vi "CRYUser Equation Parametes Table.vi"() -> ()   [LabVIEW 2013]
uses:
  Typedef Control/CRYUser Equation Cluster.ctl
  Typedef Control/CRYData Cluster Array.ctl
  Typedef Control/CRYData Cluster.ctl
  <vilib>/Utility/miscctls.llb/LVRowAndColumnTypeDef.ctl
  CRYPost Processing Global.vi
  CRYWindow/SubVI/CRYMain Sub Window Global.vi
panel:
  in  "DataNames":string[](array[string])
  in  "Curves&Values":T1 {"Z data" items=["dB", "Lin"]; "X data" items=["dB", "Lin"]; "Y data" items=["dB", "Lin"]; "Z dB ref" format="%.1f"; "Z axis" items=["Log", "Lin"]; "X dB ref" format="%.1f"; "X axis" items=["Log", "Lin"]; "Y axis" items=["Log", "Lin"]; "Y dB ref" format="%.1f"; "Curve"."z" format="%.2f"; "Curve"."y" format="%.2f"; "Curve"."x" format="%.2f"}
  in  "CurLibChange":bool caption="Add Lib"
  in  "On/Off Line":bool
  out "Clear All":bool
  out "In_Table Change":i32
  out "Res_Table Change":bool
  out "Row_unit res":i32
  out "User Equation Cluster":T3 {"Results axis" items=["x", "y", "z"]; "Input axis" items=["x", "y", "z"]; "Custom unit results array"."dB ref" format="%.2f"; "Custom unit input array"."dB ref" format="%.2f"}
  out "Load":bool
  out "String Ref Out":refnum<vi>
  out "Row_unit":i32
  in  "Unit_in":bool
  out "Row_axis":i32
  in  "Axis_Rnig":u16(ring) items=["x", "y", "z"]
  out "Row":i32
  in  "Ope_Ring":u16(ring) caption="Type" items=["<Select Operand>", "unity cal-in corr-in", "CRY33x Mic 1 corr-in", "CRY33x Mic 2 corr-in", "CRY33x Mic 3 corr-in", "CRY33x Mic 4 corr-in", "USB In L corr-in", "USB In R corr-in", "unity cal-out corr-out", "unity cal-out eq-out", "CRY602 Mouth 1 corr-out", "CRY602 Mouth 1 eq-out", "CRY602 Mouth 2 corr-out", "CRY602 Mouth 2 eq-out", "USB Out R corr-out", "USB Out R eq-out", "unity cal-in sens-in", "CRY33x Mic 1 sens-in", "CRY33x Mic 2 sens-in", "CRY33x Mic 3 sens-in", "CRY33x Mic 4 sens-in", "USB In L sens-in", "USB In R sens-in", "unity cal-out sens-out", "CRY602 Mouth 1 sens-out", "CRY602 Mouth 2 sens-out", "USB Out R sens-out", "User Defined Constant", "Remove this Item"]
  in  "stop":bool
  in  "Input_Table":string[][](table)
  in  "Unit_res":bool
  in  "Result_Table":string[][](table)
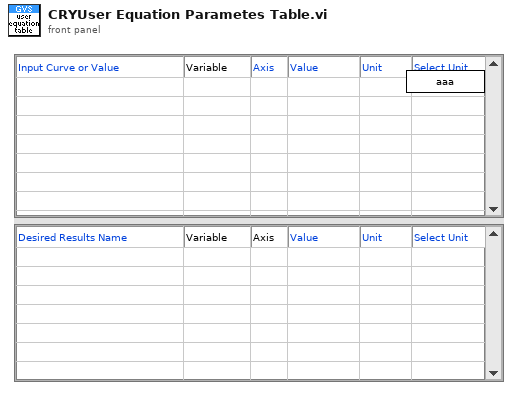
[diagram p1: front panel]
types:
  T1 = typedef "CRYData Cluster Array.ctl" = T2[]
  T2 = typedef "CRYData Cluster.ctl" = cluster{"Name":string, "Curve":cluster{"x":dbl, "y":dbl, "z":dbl}[], "X data":u16, "Y data":u16, "Z data":u16, "X axis":u16, "Y axis":u16, "Z axis":u16, "X unit":string, "Y unit":string, "Z unit":string, "X dB ref":dbl, "Y dB ref":dbl, "Z dB ref":dbl, "single val":bool, "protected":bool, "display X":bool, "display Y":bool, "display Z":bool, "Test Info":string, "Step No.":i32, "Plot Settings":cluster{"Color":u32, "Interpolation":u8, "Point Style":u8, "Line Style":u8, "Point Color":u32, "Line Width":u8, "Bar Plot Style":u8, "Fill To":i16}, "AutoProtect":bool}
  T3 = typedef "CRYUser Equation Cluster.ctl" = cluster{"Custom unit input array":cluster{"use custom":bool, "lin/log":u16, "unit":string, "dB ref":dbl, "common dB":u16}[], "Custom unit results array ":cluster{"use custom":bool, "lin/log":u16, "unit":string, "dB ref":dbl, "common dB":u16}[], "Desired Result Variables":string[], "Desired Result Names":string[], "Input Curve Names":string[], "Input Curve Variables":string[], "equation":string, "Input axis":u16[], "Results axis":u16[], "# input curves":i32, "# Desired result curves ":i32, "Input Values":string[], "Result Values":string[]}
  T4 = typedef "LVRowAndColumnTypeDef.ctl" = cluster{"Row":i32, "Column":i32}
  T5 = typedef "LVRectTypeDef.ctl" = cluster{"Left":i16, "Top":i16, "Right":i16, "Bottom":i16}
  T6 = typedef "CRYStep.ctl" = cluster{"No.VI":i32, "Category":string, "StepName":string, "Seq setup flattened":string, "Comment":string, "Steps config.":bool[], "Jump config":i32[], "Start":dbl, "Increment":dbl, "Name":string, "Unit":string, "Y data":u16, "Y prefix":string, "Y dB ref":dbl, "Y unit":string, "Repeat State Array":cluster{"Start":dbl, "Increment":dbl, "Count":i32, "Num":i32}[]}
  T7 = cluster{"use custom":bool, "lin/log":u16, "unit":string, "dB ref":dbl, "common dB":u16}
  T8 = enum16{"OK", "Yes", "YesNo", "YesNoCancel", "ReplaceAppend"}
  T9 = cluster{"use custom":bool, "lin/log":u16, "unit":string, "dB ref":dbl, "common dB":u16}[]
  T10 = typedef "LVPoint32TypeDef.ctl" = cluster{"Horizontal":i32, "Vertical":i32}
  T11 = typedef "LVBoundsTypeDef.ctl" = cluster{"Width":u32, "Height":u32}
  T12 = typedef "LVPositionTypeDef.ctl" = cluster{"Left":i32, "Top":i32}
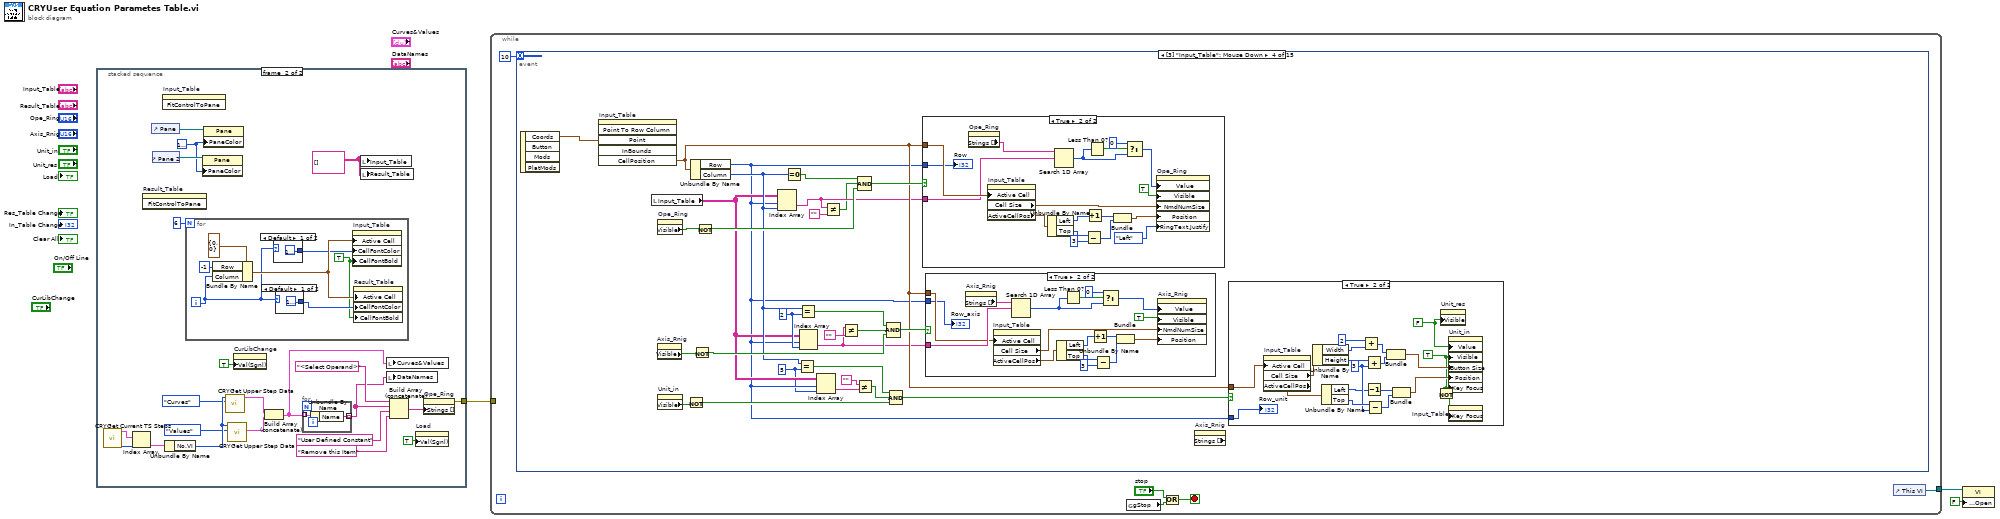
[diagram p0: block diagram]
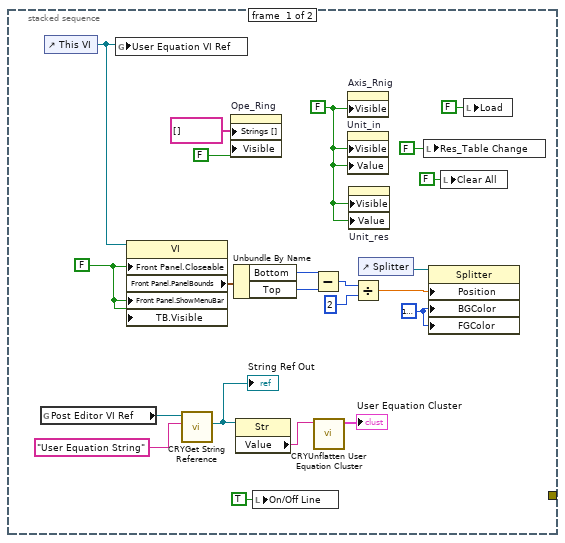
[diagram p2: hidden frame]
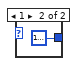
[diagram p3: hidden frame]
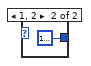
[diagram p4: hidden frame]
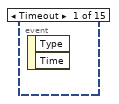
[diagram p5: hidden frame]
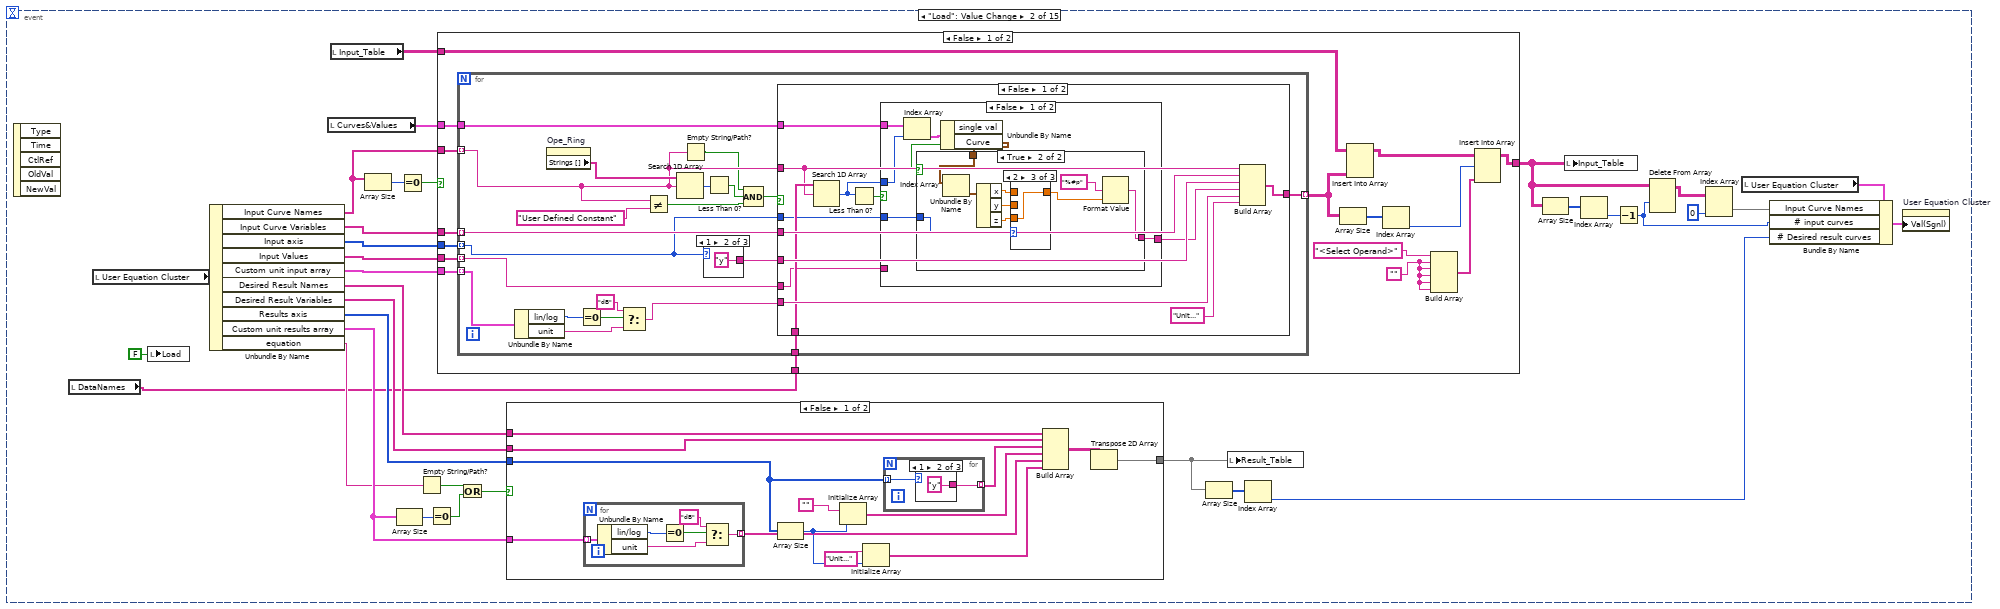
[diagram p6: hidden frame]
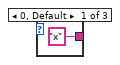
[diagram p7: hidden frame]
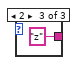
[diagram p8: hidden frame]
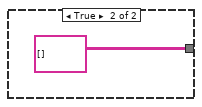
[diagram p9: hidden frame]
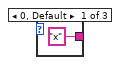
[diagram p10: hidden frame]
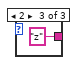
[diagram p11: hidden frame]
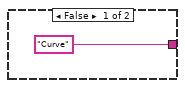
[diagram p12: hidden frame]
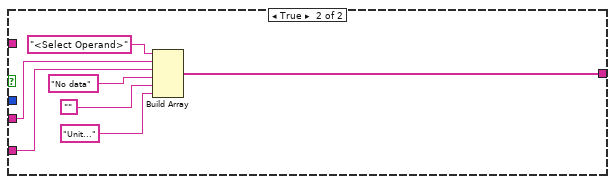
[diagram p16: hidden frame]
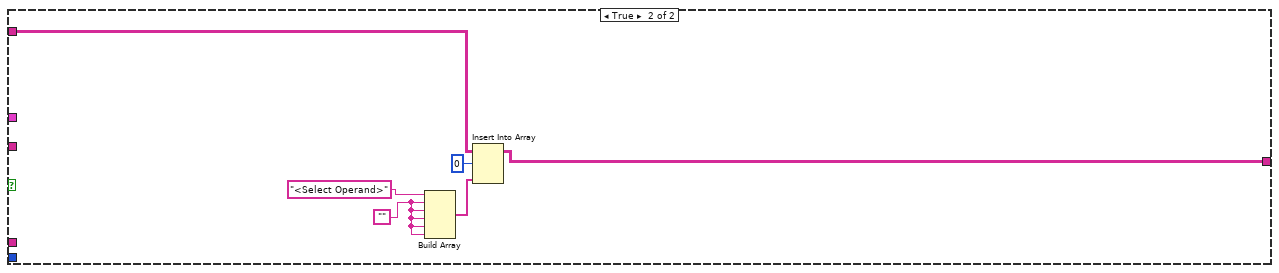
[diagram p17: hidden frame]
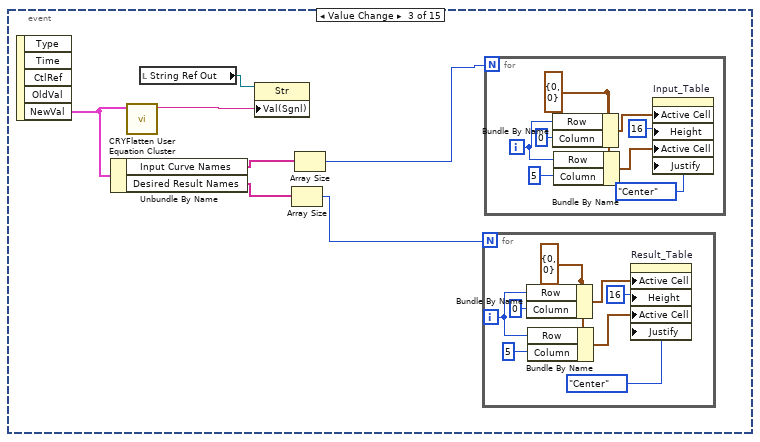
[diagram p18: hidden frame]
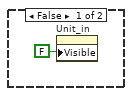
[diagram p19: hidden frame]
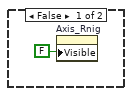
[diagram p20: hidden frame]
diagram:
  n1 = stacked-sequence {
    tunnel: [_ w26] -> w1
    frame #0 {
      w11 = u32 16777238
      w12 = FALSE ("Front Panel Window:Closeable")
      w22 = FALSE ("Visible")
      n2 = global read "CRYPost Processing Global.vi" "Post Editor VI Ref"() -> (w6:refnum<vi>)
      n3 = control-ref of="This VI"() -> (w4:refnum<vi>)
      n4 = global write "CRYPost Processing Global.vi" "User Equation VI Ref"(w4) -> ()
      n5 = property class="VI"(reference=w4, "Front Panel.Closeable"=w12, "Front Panel.ShowMenuBar"=w12, "TB.Visible"=w12) -> ("Front Panel.PanelBounds"=w18:T5)  [unwired: 1 in, 2 out]
      n6 = call "CRYGet String Reference.vi"("Label Name"="User Equation String", "VI Refnum"=w6) -> ("String Ref Out"=w8:refnum<vi>)  [unwired: 9 out]
      "String Ref Out" <- w8
      n7 = property on="Ope_Ring" class="Ring (strict)"("Strings []"=string[] [], "Visible"=FALSE) -> ()  [unwired: 2 in, 2 out]
      n8 = Unbundle By Name(w18) -> ("Bottom"=w17:i16, "Top"=w14:i16)
      n9 = property class="Str"(reference=w8) -> ("Value"=w9:string)  [unwired: 1 in, 2 out]
      n10 = local write "On/Off Line"(TRUE ("On/Off Line")) -> ()
      n11 = Subtract(x=w17, y=w14) -> (x-y=w16:i16)
      n12 = call "CRYUnflatten User Equation Cluster.vi"("Flatten user equation cluster string"=w9) -> ("User Equation Cluster"=→"User Equation Cluster":T3)  [unwired: 8 in, 2 out]
      n13 = property on="Axis_Rnig" class="Ring (strict)"("Visible"=w22) -> ()  [unwired: 2 in, 2 out]
      n14 = property on="Unit_in" class="Bool (strict)"("Visible"=w22, "Value"=w22) -> ()  [unwired: 2 in, 2 out]
      n15 = property on="Unit_res" class="Bool (strict)"("Visible"=w22, "Value"=w22) -> ()  [unwired: 2 in, 2 out]
      n16 = Divide(x=w16, y=i16 2) -> (x/y=w13:dbl)
      n17 = control-ref of="Splitter"() -> (w19:refnum<vi>)
      n18 = local write "Res_Table Change"(FALSE ("Table Change")) -> ()
      n19 = property class="Splitter"(reference=w19, "Position"=w13, "BGColor"=w11, "FGColor"=w11) -> ()  [unwired: 1 in, 2 out]
      n20 = local write "Clear All"(FALSE ("Clear All")) -> ()
      n21 = local write "Load"(FALSE ("Load")) -> ()
    }
    frame #1 {
      w38 = string[][] [] ("Result Table")
      w45 = u32 16777238
      n22 = call "CRYGet Current TS Steps.vi"() -> ("SelectStepNumber in Tree"=w34:i32, "Steps"=w33:T6[])  [unwired: 7 in, 3 out]
      n23 = Index Array(array=w33, index=w34) -> (element=w32:T6)
      n24 = invoke on="Result_Table" class="Tbl (strict)" method="FitControlToPane"() -> ()  [unwired: 3 in, 3 out]
      n25 = control-ref of="Pane"() -> (w47:refnum<vi>)
      n26 = control-ref of="Pane 2"() -> (w46:refnum<vi>)
      n27 = invoke on="Input_Table" class="Tbl (strict)" method="FitControlToPane"() -> ()  [unwired: 3 in, 3 out]
      n28 = Unbundle By Name(w32) -> ("No.VI"=w37:i32)
      n29 = for {
        N: 6 -> [_]
        i -> [w50]
        w48 = TRUE ("Active Cell:Cell Font:Bold")
        n30 = Bundle By Name(cluster=T4 {"Row"=0, "Column"=0} ("Active Cell:Active Cell"), "Row"=-1, "Column"=w50) -> (w52:T4)
        n31 = case shown="Default" w50 {
          tunnel: [u32 16777222 u32 16777222] -> w49
          frame Default {
          }
          frame 1 {
          }
        }
        n32 = case shown="Default" w50 {
          tunnel: [u32 16777222 u32 16777222] -> w51
          frame Default {
          }
          frame 1, 2 {
          }
        }
        n33 = property on="Input_Table" class="Tbl (strict)"("Active Cell"=w52, "CellFontColor"=w49, "CellFontBold"=w48) -> ()  [unwired: 2 in, 2 out]
        n34 = property on="Result_Table" class="Tbl (strict)"("Active Cell"=w52, "CellFontColor"=w51, "CellFontBold"=w48) -> ()  [unwired: 2 in, 2 out]
      }
      n35 = property class="Pane"(reference=w46, "PaneColor"=w45) -> ()  [unwired: 1 in, 2 out]
      n36 = property class="Pane"(reference=w47, "PaneColor"=w45) -> ()  [unwired: 1 in, 2 out]
      n37 = call "CRYGet Upper Step Data.vi"("Type In"=enum16{"Curves", "Values", "Results", "WFM"}."Curves", "No.VI"=w37) -> ("Curve array"=w31:T1)  [unwired: 9 out]
      n38 = call "CRYGet Upper Step Data.vi"("Type In"=enum16{"Curves", "Values", "Results", "WFM"}."Values", "No.VI"=w37) -> ("Value array"=w30:T1)  [unwired: 9 out]
      n39 = property on="CurLibChange" class="Bool (strict)"("Val(Sgnl)"=TRUE ("Value (Signaling)")) -> ()  [unwired: 2 in, 2 out]
      n40 = Build Array (concatenate)(w31, w30) -> (w27:T1)
      n41 = for {
        tunnel: w27 -> [w60] mode=indexing
        tunnel: [w59] -> w28 mode=indexing
        n42 = Unbundle By Name(w60) -> ("Name"=w59:string)
      }
      n43 = local write "Input_Table"(w38) -> ()
      n44 = local write "Result_Table"(w38) -> ()
      n45 = local write "Curves&Values"(w27) -> ()
      n46 = local write "DataNames"(w28) -> ()
      n47 = Build Array (concatenate)("<Select Operand>", w28, "User Defined Constant", "Remove this Item") -> (w41:string[])
      n48 = property on="Load" class="Bool (strict)"("Val(Sgnl)"=TRUE ("Value (Signaling)")) -> ()  [unwired: 2 in, 2 out]
      n49 = property on="Ope_Ring" class="Ring (strict)"("Strings []"=w41) -> (error out=w26:errorcluster)  [unwired: 2 in, 1 out]
    }
  }
  n50 = while {
    tunnel: [w61] -> w2
    tunnel: w1 -> [_]
    stop <- w62 stop-if-true
    n51 = event shown="[3] \"Input_Table\": Mouse Down" {
      selector: _ -> [_ _ _ _ _ _ _ _ _ _ _ _ _ _ _]
      dyn-events: _ -> [_ _ _ _ _ _ _ _ _ _ _ _ _ _ _]
      timeout: 10 -> [_ _ _ _ _ _ _ _ _ _ _ _ _ _ _]
      event Timeout {
        n52 = event-data() -> ()  [unwired: 1 in, 2 out]
      }
      event "Load": Value Change {
        n53 = event-data() -> ()  [unwired: 1 in, 5 out]
        n54 = local read "DataNames"() -> (w66:string[])
        n55 = local read "User Equation Cluster"() -> (w98:T3)
        n56 = local write "Load"(FALSE ("Load")) -> ()
        n57 = Unbundle By Name(w98) -> ("Input Curve Names"=w93:string[], "Input Curve Variables"=w90:string[], "Input axis"=w89:u16[], "Input Values"=w88:string[], "Custom unit input array"=w87:T9, "Desired Result Names"=w96:string[], "Desired Result Variables"=w95:string[], "Results axis"=w94:u16[], "Custom unit results array"=w77:T9, "equation"=w69:string)
        n58 = local read "Curves&Values"() -> (w67:T1)
        n59 = local read "Input_Table"() -> (w91:string[][])
        n60 = Array Size(array=w93) -> (size(s)=w92:i32)
        n61 = Array Size(array=w77) -> (size(s)=w76:i32)
        n62 = Equal To 0?(x=w92) -> (x = 0?=w78:bool)
        n63 = Empty String/Path?(string/path=w69) -> (empty?=w68:bool)
        n64 = Equal To 0?(x=w76) -> (x = 0?=w75:bool)
        n65 = case shown="False" w78 {
          tunnel: w93 -> [w139 _]
          tunnel: w91 -> [w138 w206]
          tunnel: w90 -> [w137 _]
          tunnel: w89 -> [w136 _]
          tunnel: w88 -> [w135 _]
          tunnel: w87 -> [w134 _]
          tunnel: [w133 w205] -> w80
          tunnel: w66 -> [w125 _]
          tunnel: w67 -> [w124 _]
          frame False {
            w132 = ""
            n66 = for {
              tunnel: w139 -> [w145] mode=indexing
              tunnel: w137 -> [w156] mode=indexing
              tunnel: w136 -> [w140] mode=indexing
              tunnel: w135 -> [w153] mode=indexing
              tunnel: w134 -> [w148] mode=indexing
              tunnel: [w154] -> w130 mode=indexing
              tunnel: w125 -> [w142]
              tunnel: w124 -> [w141]
              n67 = Unbundle By Name(w148) -> ("lin/log"=w149:u16, "unit"=w151:string)
              n68 = property on="Ope_Ring" class="Ring (strict)"() -> ("Strings []"=w146:string[])  [unwired: 2 in, 2 out]
              n69 = Equal To 0?(x=w149) -> (x = 0?=w150:bool)
              n70 = Select(t="dB", s=w150, f=w151) -> (s? t:f=w147:string)
              n71 = Not Equal?(x=w145, y="User Defined Constant") -> (x != y?=w158:bool)
              n72 = Search 1D Array(1D array=w146, element=w145) -> (index of element=w160:i32)  [unwired: 1 in]
              n73 = Empty String/Path?(string/path=w145) -> (empty?=w144:bool)
              n74 = case shown="1" w140 {
                tunnel: ["x" "y" "z"] -> w155
                frame 0, Default {
                }
                frame 1 {
                }
                frame 2 {
                }
              }
              n75 = Less Than 0?(x=w160) -> (x < 0?=w159:bool)
              n76 = Compound Arithmetic op=AND(w144, w159, w158) -> (w157:bool)
              n77 = case shown="False" w157 {
                tunnel: w156 -> [w176 w203]
                tunnel: w155 -> [w175 w202]
                tunnel: [w172 w198] -> w154
                tunnel: w145 -> [w170 _]
                tunnel: w153 -> [w168 _]
                tunnel: w147 -> [w174 _]
                tunnel: w142 -> [w171 _]
                tunnel: w141 -> [w165 _]
                tunnel: w140 -> [w164 _]
                frame False {
                  n78 = Search 1D Array(1D array=w171, element=w170) -> (index of element=w166:i32)  [unwired: 1 in]
                  n79 = Less Than 0?(x=w166) -> (x < 0?=w169:bool)
                  n80 = case shown="False" w169 {
                    tunnel: w168 -> [_ w197]
                    tunnel: [w179 w197] -> w167
                    tunnel: w166 -> [w182 _]
                    tunnel: w165 -> [w183 _]
                    tunnel: w164 -> [w178 _]
                    frame False {
                      n81 = Index Array(array=w183, index=w182) -> (element=w181:T2)
                      n82 = Unbundle By Name(w181) -> ("single val"=w180:bool, "Curve"=w177:cluster{"x":dbl, "y":dbl, "z":dbl}[])
                      n83 = case shown="True" w180 {
                        tunnel: ["Curve" ("output string") w185] -> w179
                        tunnel: w178 -> [_ w192]
                        tunnel: w177 -> [_ w193]
                        frame False {
                        }
                        frame True {
                          n84 = Index Array(array=w193) -> (element=w191:cluster{"x":dbl, "y":dbl, "z":dbl})  [unwired: 1 in]
                          n85 = Unbundle By Name(w191) -> ("x"=w190:dbl, "y"=w189:dbl, "z"=w188:dbl)
                          n86 = case shown="2" w192 {
                            tunnel: w190 -> [w194 _ _]
                            tunnel: w189 -> [_ w195 _]
                            tunnel: w188 -> [_ _ w196]
                            tunnel: [w194 w195 w196] -> w186
                            frame 0, Default {
                            }
                            frame 1 {
                            }
                            frame 2 {
                            }
                          }
                          n87 = Format Value(format string="%#p", value (0)=w186) -> (output string=w185:string)  [unwired: 1 in]
                        }
                      }
                    }
                    frame True {
                    }
                  }
                  n88 = Build Array(w170, w176, w175, w167, w174, "Unit..." ("element")) -> (w172:string[])
                }
                frame True {
                  n89 = Build Array("<Select Operand>", w203, w202, "No data" ("element"), "", "Unit..." ("element")) -> (w198:string[])
                }
              }
            }
            n90 = Array Size(array=w130) -> (size(s)=w129:i32[])
            n91 = Insert Into Array(array=w138, new element=w130) -> (w128:string[][])  [unwired: 2 in]
            n92 = Index Array(array=w129) -> (element=w127:i32)  [unwired: 1 in]
            n93 = Build Array("<Select Operand>", w132, w132, w132, w132, w132) -> (w126:string[])
            n94 = Insert Into Array(array=w128, index (row)=w127, new element=w126) -> (w133:string[][])  [unwired: 1 in]
          }
          frame True {
            w210 = ""
            n95 = Build Array("<Select Operand>", w210, w210, w210, w210, w210) -> (w207:string[])
            n96 = Insert Into Array(array=w206, index (row)=0, new element=w207) -> (w205:string[][])  [unwired: 1 in]
          }
        }
        n97 = Or(x=w68, y=w75) -> (x .or. y?=w74:bool)
        n98 = case shown="False" w74 {
          tunnel: w96 -> [w111 _]
          tunnel: w95 -> [w110 _]
          tunnel: w94 -> [w109 _]
          tunnel: [w100 string[][] []] -> w71
          tunnel: w77 -> [w99 _]
          frame False {
            n99 = for {
              tunnel: w99 -> [w117] mode=indexing
              tunnel: [w112] -> w104 mode=indexing
              n100 = Unbundle By Name(w117) -> ("lin/log"=w116:u16, "unit"=w114:string)
              n101 = Equal To 0?(x=w116) -> (x = 0?=w115:bool)
              n102 = Select(t="dB", s=w115, f=w114) -> (s? t:f=w112:string)
            }
            n103 = Array Size(array=w109) -> (size(s)=w102:i32)
            n104 = Initialize Array("" ("element"), w102) -> (w105:string[])
            n105 = Initialize Array("Unit..." ("element"), w102) -> (w101:string[])
            n106 = for {
              tunnel: w109 -> [w119] mode=indexing
              tunnel: [w118] -> w107 mode=indexing
              n107 = case shown="1" w119 {
                tunnel: ["x" "y" "z"] -> w118
                frame 0, Default {
                }
                frame 1 {
                }
                frame 2 {
                }
              }
            }
            n108 = Build Array(w111, w110, w107, w105, w104, w101) -> (w108:string[][])
            n109 = Transpose 2D Array(2D array=w108) -> (transposed array=w100:string[][])
          }
          frame True {
          }
        }
        n110 = Array Size(array=w71) -> (size(s)=w72:i32[])
        n111 = local write "Result_Table"(w71) -> ()
        n112 = Index Array(array=w72) -> (element=w70:i32)  [unwired: 1 in]
        n113 = Array Size(array=w80) -> (size(s)=w82:i32[])
        n114 = local write "Input_Table"(w80) -> ()
        n115 = Index Array(array=w82) -> (element=w81:i32)  [unwired: 1 in]
        n116 = Decrement(x=w81) -> (x-1=w73:i32)
        n117 = Delete From Array(array=w80, index (row)=w73) -> (array with subset deleted=w79:string[][])  [unwired: 2 in, 1 out]
        n118 = Index Array(array=w79, index (col)=0 ("disabled index (col)")) -> (element=w83:string[])  [unwired: 1 in]
        n119 = local read "User Equation Cluster"() -> (w85:T3)
        n120 = Bundle By Name(cluster=w85, "Input Curve Names"=w83, "# input curves"=w73, "# Desired result curves"=w70) -> (w84:T3)
        n121 = property on="User Equation Cluster" class="Clust (strict)"("Val(Sgnl)"=w84) -> ()  [unwired: 2 in, 2 out]
      }
      event Value Change {
        n122 = event-data() -> ("NewVal"=w215:T3)  [unwired: 1 in, 4 out]
        n123 = Unbundle By Name(w215) -> ("Input Curve Names"=w214:string[], "Desired Result Names"=w212:string[])
        n124 = call "CRYFlatten User Equation Cluster.vi"("user equation cluster"=w215) -> ("Flatten String"=w216:string)  [unwired: 10 in]
        n125 = local read "String Ref Out"() -> (w217:refnum<vi>)
        n126 = property class="Str"(reference=w217, "Val(Sgnl)"=w216) -> ()  [unwired: 1 in, 2 out]
        n127 = Array Size(array=w212) -> (size(s)=w211:i32)
        n128 = Array Size(array=w214) -> (size(s)=w213:i32)
        n129 = for {
          N: w211 -> [_]
          i -> [w221]
          w222 = T4 {"Row"=0, "Column"=0} ("Active Cell:Active Cell")
          n130 = Bundle By Name(cluster=w222, "Row"=w221, "Column"=0) -> (w225:T4)
          n131 = Bundle By Name(cluster=w222, "Row"=w221, "Column"=5) -> (w219:T4)
          n132 = property on="Result_Table" class="Tbl (strict)"("Active Cell"=w225, "Height"=u32 16 ("Active Cell:Cell Size:Height"), "Active Cell"=w219, "Justify"=enum16{"Left", "Center", "Right"}."Center" ("Active Cell:Cell Justification")) -> ()  [unwired: 2 in, 2 out]
        }
        n133 = for {
          N: w213 -> [_]
          i -> [w229]
          w230 = T4 {"Row"=0, "Column"=0} ("Active Cell:Active Cell")
          n134 = Bundle By Name(cluster=w230, "Row"=w229, "Column"=0) -> (w232:T4)
          n135 = Bundle By Name(cluster=w230, "Row"=w229, "Column"=5) -> (w227:T4)
          n136 = property on="Input_Table" class="Tbl (strict)"("Active Cell"=w232, "Height"=u32 16 ("Active Cell:Cell Size:Height"), "Active Cell"=w227, "Justify"=enum16{"Left", "Center", "Right"}."Center" ("Active Cell:Cell Justification")) -> ()  [unwired: 2 in, 2 out]
        }
      }
      event "Input_Table": Mouse Down {
        w237 = 5 ("y")
        w256 = 2 ("y")
        n137 = event-data() -> ("Coords"=w259:T10)  [unwired: 1 in, 3 out]
        n138 = invoke on="Input_Table" class="Tbl (strict)" method="Point To Row Column"("Point"=w259) -> ("CellPosition"=w246:T4)  [unwired: 5 in, 5 out]
        n139 = local read "Input_Table"() -> (w239:string[][])
        n140 = property on="Axis_Rnig" class="Ring (strict)"() -> ("Visible"=w254:bool)  [unwired: 2 in, 2 out]
        n141 = property on="Ope_Ring" class="Ring (strict)"() -> ("Visible"=w258:bool)  [unwired: 2 in, 2 out]
        n142 = property on="Unit_in" class="Bool (strict)"() -> ("Visible"=w251:bool)  [unwired: 2 in, 2 out]
        n143 = Not(x=w251) -> (.not. x?=w248:bool)
        n144 = Unbundle By Name(w246) -> ("Row"=w238:i32, "Column"=w250:i32)
        n145 = Not(x=w254) -> (.not. x?=w253:bool)
        n146 = Not(x=w258) -> (.not. x?=w257:bool)
        n147 = Index Array(array=w239, index (row)=w238, index (col)=w250) -> (element=w245:string)
        n148 = Equal To 0?(x=w250) -> (x = 0?=w261:bool)
        n149 = Equal?(x=w250, y=w237) -> (x = y?=w249:bool)
        n150 = Equal?(x=w250, y=w256) -> (x = y?=w255:bool)
        n151 = Index Array(array=w239, index (row)=w238, index (col)=w256) -> (element=w241:string)
        n152 = Index Array(array=w239, index (row)=w238, index (col)=w237) -> (element=w235:string)
        n153 = Not Equal?(x=w245, y="") -> (x != y?=w243:bool)
        n154 = Not Equal?(x=w241, y="") -> (x != y?=w240:bool)
        n155 = Not Equal?(x="", y=w235) -> (x != y?=w234:bool)
        n156 = Compound Arithmetic op=AND(w261, w243, w257) -> (w260:bool)
        n157 = Compound Arithmetic op=AND(w255, w240, w253) -> (w252:bool)
        n158 = Compound Arithmetic op=AND(w249, w234, w248) -> (w247:bool)
        n159 = case shown="True" w260 {
          tunnel: w246 -> [_ w315]
          tunnel: w245 -> [_ w309]
          tunnel: w238 -> [_ w307]
          frame False {
            n160 = property on="Ope_Ring" class="Ring (strict)"("Visible"=FALSE) -> ()  [unwired: 2 in, 2 out]
          }
          frame True {
            n161 = property on="Ope_Ring" class="Ring (strict)"() -> ("Strings []"=w310:string[])  [unwired: 2 in, 2 out]
            n162 = property on="Input_Table" class="Tbl (strict)"("Active Cell"=w315) -> ("Cell Size"=w302:T11, "ActiveCellPos"=w314:T12)  [unwired: 2 in, 2 out]
            n163 = Unbundle By Name(w314) -> ("Left"=w303:i32, "Top"=w305:i32)
            n164 = Search 1D Array(1D array=w310, element=w309) -> (index of element=w312:i32)  [unwired: 1 in]
            n165 = Subtract(x=w305, y=3) -> (x-y=w304:i32)
            n166 = Increment(x=w303) -> (x+1=w301:i32)
            n167 = Less Than 0?(x=w312) -> (x < 0?=w313:bool)
            n168 = Bundle(w301, w304) -> (w316:cluster{i32, i32})  [unwired: 1 in]
            n169 = Select(t=0, s=w313, f=w312) -> (s? t:f=w308:i32)
            n170 = property on="Ope_Ring" class="Ring (strict)"("Value"=w308, "Visible"=TRUE, "NmdNumSize"=w302, "Position"=w316, "RingText.Justify"=enum16{"Left", "Center", "Right"}."Left" ("Ring Text.Justification")) -> ()  [unwired: 2 in, 2 out]
            "Row" <- w307
          }
        }
        n171 = case shown="True" w252 {
          tunnel: w246 -> [_ w297]
          tunnel: w241 -> [_ w299]
          tunnel: w238 -> [_ w290]
          frame False {
            n172 = property on="Axis_Rnig" class="Ring (strict)"("Visible"=FALSE) -> ()  [unwired: 2 in, 2 out]
          }
          frame True {
            n173 = property on="Axis_Rnig" class="Ring (strict)"() -> ("Strings []"=w283:string[])  [unwired: 2 in, 2 out]
            n174 = property on="Input_Table" class="Tbl (strict)"("Active Cell"=w297) -> ("Cell Size"=w296:T11, "ActiveCellPos"=w292:T12)  [unwired: 2 in, 2 out]
            n175 = Search 1D Array(1D array=w283, element=w299) -> (index of element=w287:i32)  [unwired: 1 in]
            n176 = Unbundle By Name(w292) -> ("Left"=w285:i32, "Top"=w293:i32)
            n177 = Less Than 0?(x=w287) -> (x < 0?=w288:bool)
            n178 = Increment(x=w285) -> (x+1=w284:i32)
            n179 = Subtract(x=w293, y=3) -> (x-y=w295:i32)
            n180 = Select(t=0, s=w288, f=w287) -> (s? t:f=w286:i32)
            n181 = Bundle(w284, w295) -> (w291:cluster{i32, i32})  [unwired: 1 in]
            n182 = property on="Axis_Rnig" class="Ring (strict)"("Value"=w286, "Visible"=TRUE, "NmdNumSize"=w296, "Position"=w291) -> ()  [unwired: 2 in, 2 out]
            "Row_axis" <- w290
          }
        }
        n183 = property on="Axis_Rnig" class="Ring (strict)" props=["Strings []"]() -> ()  [unwired: 2 in, 3 out]
        n184 = case shown="True" w247 {
          tunnel: w246 -> [_ w280]
          tunnel: w238 -> [_ w274]
          frame False {
            n185 = property on="Unit_in" class="Bool (strict)"("Visible"=FALSE) -> ()  [unwired: 2 in, 2 out]
          }
          frame True {
            w270 = FALSE ("Unit")
            w272 = u32 3 ("y")
            w264 = TRUE ("Visible")
            n186 = property on="Input_Table" class="Tbl (strict)"("Active Cell"=w280) -> ("Cell Size"=w278:T11, "ActiveCellPos"=w281:T12)  [unwired: 2 in, 2 out]
            n187 = Unbundle By Name(w278) -> ("Width"=w266:u32, "Height"=w276:u32)
            n188 = Unbundle By Name(w281) -> ("Left"=w269:i32, "Top"=w273:i32)
            n189 = Add(x=u32 2, y=w266) -> (x+y=w267:u32)
            n190 = Add(x=w276, y=w272) -> (x+y=w277:u32)
            n191 = Decrement(x=w269) -> (x-1=w268:i32)
            n192 = Subtract(x=w273, y=w272) -> (x-y=w271:u32)
            n193 = Bundle(w267, w277) -> (w275:cluster{u32, u32})  [unwired: 1 in]
            n194 = Bundle(w268, w271) -> (w279:cluster{i32, u32})  [unwired: 1 in]
            n195 = Not(x=w264) -> (.not. x?=w263:bool)
            n196 = property on="Unit_res" class="Bool (strict)"("Visible"=w270) -> ()  [unwired: 2 in, 2 out]
            n197 = property on="Unit_in" class="Bool (strict)"("Value"=w270, "Visible"=w264, "Button Size"=w275, "Position"=w279, "Key Focus"=w264) -> ()  [unwired: 2 in, 2 out]
            n198 = property on="Input_Table" class="Tbl (strict)"("Key Focus"=w263) -> ()  [unwired: 2 in, 2 out]
            "Row_unit" <- w274
          }
        }
      }
      event "Ope_Ring": Value Change {
        w369 = ""
        w322 = "User Defined Constant"
        w345 = "<Select Operand>"
        n199 = event-data() -> ()  [unwired: 1 in, 5 out]
        n200 = local read "Input_Table"() -> (w337:string[][])
        n201 = property on="Ope_Ring" class="Ring (strict)"("Visible"=FALSE) -> ("RingText.Text"=w366:string)  [unwired: 2 in, 2 out]
        n202 = local read "Row"() -> (w336:i32)
        n203 = Index Array(array=w337, index (row)=w336) -> (element=w338:string[])  [unwired: 1 in]
        n204 = Delete From Array(array=w338, index=0) -> (array with subset deleted=w340:string[])  [unwired: 1 in, 1 out]
        n205 = Equal?(x=w366, y=w345) -> (x = y?=w376:bool)
        n206 = for {
          tunnel: w340 -> [w382] mode=indexing
          tunnel: [w381] -> w341 mode=indexing
          n207 = Equal?(x="", y=w382) -> (x = y?=w381:bool)
        }
        n208 = Equal?(x=w366, y=w322) -> (x = y?=w375:bool)
        n209 = Equal?(x=w366, y="Remove this Item") -> (x = y?=w374:bool)
        n210 = Bundle(w376, w375, w374) -> (w373:cluster{bool, bool, bool})  [unwired: 1 in]
        n211 = local read "Curves&Values"() -> (w320:T1)
        n212 = local read "DataNames"() -> (w319:string[])
        n213 = Cluster To Array(cluster=w373) -> (array=w372:bool[])
        n214 = Search 1D Array(1D array=w341, element=FALSE) -> (index of element=w343:i32)  [unwired: 1 in]
        n215 = Search 1D Array(1D array=w372, element=TRUE) -> (index of element=w370:i32)  [unwired: 1 in]
        n216 = Less Than 0?(x=w343) -> (x < 0?=w335:bool)
        n217 = case shown="Default" w370 {
          tunnel: w366 -> [w442 w466 _]
          tunnel: w336 -> [w413 w461 w493]
          tunnel: w337 -> [w415 w462 w494]
          tunnel: [w412 w460 w492] -> w324
          tunnel: w335 -> [w410 w458 _]
          tunnel: w320 -> [w409 _ _]
          tunnel: w319 -> [w408 _ _]
          frame Default {
            n218 = Index Array(array=w415, index (row)=w413, index (col)=1 ("disabled index (col)")) -> (element=w417:string)
            n219 = Index Array(array=w415, index (col)=1 ("disabled index (col)")) -> (element=w411:string[])  [unwired: 1 in]
            n220 = for {
              tunnel: w411 -> [w452] mode=indexing
              tunnel: [w451] -> w437 mode=indexing
              n221 = Equal?(x="", y=w452) -> (x = y?=w451:bool)
            }
            n222 = for {
              tunnel: w411 -> [w457] mode=indexing
              tunnel: [w454] -> w440 mode=indexing
              n223 = Match Pattern(string=w457, regular expression="a") -> (after substring=w455:string)  [unwired: 1 in, 3 out]
              n224 = Decimal String To Number(string=w455) -> (number=w454:i32)  [unwired: 2 in, 1 out]
            }
            n225 = Search 1D Array(1D array=w408, element=w442) -> (index of element=w444:i32)  [unwired: 1 in]
            n226 = Index Array(array=w409, index=w444) -> (element=w443:T2)
            n227 = Unbundle By Name(w443) -> ("single val"=w428:bool, "Curve"=w427:cluster{"x":dbl, "y":dbl, "z":dbl}[], "Y data"=w425:u16, "Y unit"=w423:string)
            n228 = Search 1D Array(1D array=w437, element=FALSE) -> (index of element=w439:i32)  [unwired: 1 in]
            n229 = Array Max & Min(array=w440) -> (max value=w435:i32)  [unwired: 3 out]
            n230 = Increment(x=w435) -> (x+1=w434:i32)
            n231 = Less Than 0?(x=w439) -> (x < 0?=w436:bool)
            n232 = case shown="True" w428 {
              tunnel: w427 -> [_ w450]
              tunnel: ["Curve" ("output string") w446] -> w426
              frame False {
              }
              frame True {
                n233 = Index Array(array=w450) -> (element=w449:cluster{"x":dbl, "y":dbl, "z":dbl})  [unwired: 1 in]
                n234 = Unbundle By Name(w449) -> ("y"=w448:dbl)
                n235 = Format Value(format string="%#p", value (0)=w448) -> (output string=w446:string)  [unwired: 1 in]
              }
            }
            n236 = Select(t=0 ("index of element"), s=w436, f=w434) -> (s? t:f=w432:i32)
            n237 = Number To Decimal String(number=w432) -> (decimal integer string=w431:string)  [unwired: 1 in]
            n238 = Equal To 0?(x=w425) -> (x = 0?=w424:bool)
            n239 = Concatenate Strings("a" ("string"), w431) -> (w418:string)
            n240 = Select(t="dB", s=w424, f=w423) -> (s? t:f=w421:string)
            n241 = Select(t=w418, s=w410, f=w417) -> (s? t:f=w416:string)
            n242 = Build Array(w442, w416, "y" ("element"), w426, w421, "Unit..." ("element")) -> (w414:string[])
            n243 = Replace Array Subset(array=w415, new element=w414, index (row)=w413) -> (w412:string[][])  [unwired: 1 in]
          }
          frame 1 {
            n244 = Index Array(array=w462, index (row)=w461, index (col)=1 ("disabled index (col)")) -> (element=w468:string)
            n245 = Index Array(array=w462, index (col)=1 ("disabled index (col)")) -> (element=w459:string[])  [unwired: 1 in]
            n246 = for {
              tunnel: w459 -> [w491] mode=indexing
              tunnel: [w488] -> w483 mode=indexing
              n247 = Match Pattern(string=w491, regular expression="a") -> (after substring=w489:string)  [unwired: 1 in, 3 out]
              n248 = Decimal String To Number(string=w489) -> (number=w488:i32)  [unwired: 2 in, 1 out]
            }
            n249 = for {
              tunnel: w459 -> [w486] mode=indexing
              tunnel: [w485] -> w480 mode=indexing
              n250 = Equal?(x="", y=w486) -> (x = y?=w485:bool)
            }
            n251 = Array Max & Min(array=w483) -> (max value=w478:i32)  [unwired: 3 out]
            n252 = Search 1D Array(1D array=w480, element=FALSE) -> (index of element=w482:i32)  [unwired: 1 in]
            n253 = Increment(x=w478) -> (x+1=w477:i32)
            n254 = Less Than 0?(x=w482) -> (x < 0?=w479:bool)
            n255 = Select(t=0 ("index of element"), s=w479, f=w477) -> (s? t:f=w475:i32)
            n256 = Number To Decimal String(number=w475) -> (decimal integer string=w474:string)  [unwired: 1 in]
            n257 = Concatenate Strings("a" ("string"), w474) -> (w469:string)
            n258 = Select(t=w469, s=w458, f=w468) -> (s? t:f=w467:string)
            n259 = Build Array(w466, w467, "y" ("element"), "Enter Value" ("element"), "Enter Unit" ("element"), "Unit..." ("element")) -> (w463:string[])
            n260 = Replace Array Subset(array=w462, new element=w463, index (row)=w461) -> (w460:string[][])  [unwired: 1 in]
          }
          frame 0, 2 {
            n261 = Delete From Array(array=w494, index (row)=w493) -> (array with subset deleted=w492:string[][])  [unwired: 2 in, 1 out]
          }
        }
        n262 = Array Size(array=w324) -> (size(s)=w359:i32[])
        n263 = Index Array(array=w359) -> (element=w358:i32)  [unwired: 1 in]
        n264 = Build Array(w345, w369, w369, w369, w369, w369) -> (w368:string[])
        n265 = Decrement(x=w358) -> (x-1=w344:i32)
        n266 = Delete From Array(array=w324, index (row)=w344) -> (array with subset deleted=w325:string[][])  [unwired: 2 in, 1 out]
        n267 = Index Array(array=w324, index (row)=w344) -> (element=w330:string[])  [unwired: 1 in]
        n268 = Index Array(array=w324, index (row)=w344, index (col)=0 ("disabled index (col)")) -> (element=w346:string)
        n269 = Delete From Array(array=w330, index=0) -> (array with subset deleted=w331:string[])  [unwired: 1 in, 1 out]
        n270 = Equal?(x=w346, y=w345) -> (x = y?=w327:bool)
        n271 = for {
          tunnel: w331 -> [w379] mode=indexing
          tunnel: [w378] -> w332 mode=indexing
          n272 = Equal?(x="", y=w379) -> (x = y?=w378:bool)
        }
        n273 = Search 1D Array(1D array=w332, element=FALSE) -> (index of element=w334:i32)  [unwired: 1 in]
        n274 = Less Than 0?(x=w334) -> (x < 0?=w328:bool)
        n275 = And(x=w327, y=w328) -> (x .and. y?=w326:bool)
        n276 = case shown="True" w326 {
          tunnel: w324 -> [w405 w407]
          tunnel: [w402 w407] -> w348
          tunnel: w368 -> [w403 _]
          frame False {
            n277 = Array Size(array=w405) -> (size(s)=w406:i32[])
            n278 = Index Array(array=w406) -> (element=w404:i32)  [unwired: 1 in]
            n279 = Insert Into Array(array=w405, index (row)=w404, new element=w403) -> (w402:string[][])  [unwired: 1 in]
          }
          frame True {
          }
        }
        n280 = Select(t=w325, s=w326, f=w324) -> (s? t:f=w357:string[][])
        n281 = Index Array(array=w357, index (col) #1=0 ("disabled index (col)"), index (col) #2=1 ("index (col)"), index (col) #3=2 ("index (col)"), index (col) #4=3 ("index (col)"), index (col) #5=4 ("index (col)")) -> (element #1=w321:string[], element #2=w355:string[], element #3=w353:string[], element #4=w351:string[], element #5=w349:string[])  [unwired: 5 in]
        n282 = local write "Input_Table"(w348) -> ()
        n283 = for {
          tunnel: w349 -> [w390] mode=indexing
          tunnel: T7 {"use custom"=FALSE, "lin/log"=0, "unit"="", "dB ref"=0.0, "common dB"=0} ("Custom unit info") -> [w396]
          tunnel: [w388] -> w361 mode=indexing
          tunnel: w322 -> [w387]
          tunnel: w321 -> [w386] mode=indexing
          n284 = Equal?(x=w386, y=w387) -> (x = y?=w385:bool)
          n285 = Equal?(x="dB", y=w390) -> (x = y?=w392:bool)
          n286 = Select(t="", s=w385, f=w390) -> (s? t:f=w389:string)
          n287 = Select(t=u16 0 ("lin/log"), s=w392, f=u16 1) -> (s? t:f=w393:u16)
          n288 = Bundle By Name(cluster=w396, "lin/log"=w393, "unit"=w389) -> (w388:T7)
        }
        n289 = for {
          tunnel: w353 -> [w398] mode=indexing
          tunnel: [w397] -> w363 mode=indexing
          n290 = case shown="\"x\", Default" w398 {
            tunnel: [0 ("disabled index (col)") 1 ("disabled index (col)") 2 ("disabled index (col)")] -> w397
            frame "x", Default {
            }
            frame "y" {
            }
            frame "z" {
            }
          }
        }
        n291 = Array Size(array=w321) -> (size(s)=w323:i32)
        n292 = local read "User Equation Cluster"() -> (w364:T3)
        n293 = Bundle By Name(cluster=w364, "# input curves"=w323, "Input Curve Names"=w321, "Input Curve Variables"=w355, "Input axis"=w363, "Input Values"=w351, "Custom unit input array"=w361) -> (w360:T3)
        n294 = property on="User Equation Cluster" class="Clust (strict)"("Val(Sgnl)"=w360) -> ()  [unwired: 2 in, 2 out]
      }
      event "Axis_Rnig": Value Change {
        n295 = event-data() -> ()  [unwired: 1 in, 5 out]
        n296 = local read "Input_Table"() -> (w499:string[][])
        n297 = local read "Row_axis"() -> (w517:i32)
        n298 = property on="Axis_Rnig" class="Ring (strict)"("Visible"=FALSE) -> ("RingText.Text"=w519:string)  [unwired: 2 in, 2 out]
        n299 = Index Array(array=w499, index (row)=w517, index (col)=0 ("disabled index (col)")) -> (element=w506:string)
        n300 = local read "DataNames"() -> (w496:string[])
        n301 = Equal?(x=w506, y="User Defined Constant") -> (x = y?=w520:bool)
        n302 = local read "Curves&Values"() -> (w495:T1)
        n303 = Select(t="y", s=w520, f=w519) -> (s? t:f=w521:string)
        n304 = Search 1D Array(1D array=w496, element=w506) -> (index of element=w507:i32)  [unwired: 1 in]
        n305 = Replace Array Subset(array=w499, new element=w521, index (row)=w517, index (col)=2 ("disabled index (col)")) -> (w518:string[][])
        n306 = Index Array(array=w495, index=w507) -> (element=w505:T2)
        n307 = case shown="False" w520 {
          tunnel: w519 -> [w544 _]
          tunnel: w518 -> [w551 w574]
          tunnel: w517 -> [w543 _]
          tunnel: [w542 w574] -> w500
          tunnel: w505 -> [w541 _]
          frame False {
            n308 = Unbundle By Name(w541) -> ("single val"=w548:bool, "Curve"=w546:cluster{"x":dbl, "y":dbl, "z":dbl}[])
            n309 = case shown="\"y\"" w544 {
              tunnel: w541 -> [w569 w571 w573]
              tunnel: [w568 w570 w572] -> w549
              frame "x", Default {
                n310 = Unbundle By Name(w569) -> ("X unit"=w568:string)
              }
              frame "y" {
                n311 = Unbundle By Name(w571) -> ("Y unit"=w570:string)
              }
              frame "z" {
                n312 = Unbundle By Name(w573) -> ("Z unit"=w572:string)
              }
            }
            n313 = Index Array(array=w546) -> (element=w545:cluster{"x":dbl, "y":dbl, "z":dbl})  [unwired: 1 in]
            n314 = Replace Array Subset(array=w551, new element=w549, index (row)=w543, index (col)=4 ("disabled index (col)")) -> (w547:string[][])
            n315 = case shown="True" w548 {
              tunnel: w547 -> [w552 w557]
              tunnel: w545 -> [_ w560]
              tunnel: w544 -> [_ w561]
              tunnel: w543 -> [_ w556]
              tunnel: [w552 w553] -> w542
              frame False {
              }
              frame True {
                n316 = case shown="\"x\", Default" w561 {
                  tunnel: w560 -> [w563 w565 w567]
                  tunnel: [w562 w564 w566] -> w559
                  frame "x", Default {
                    n317 = Unbundle By Name(w563) -> ("x"=w562:dbl)
                  }
                  frame "y" {
                    n318 = Unbundle By Name(w565) -> ("y"=w564:dbl)
                  }
                  frame "z" {
                    n319 = Unbundle By Name(w567) -> ("z"=w566:dbl)
                  }
                }
                n320 = Format Value(format string="%#p", value (0)=w559) -> (output string=w554:string)  [unwired: 1 in]
                n321 = Replace Array Subset(array=w557, new element=w554, index (row)=w556, index (col)=3 ("disabled index (col)")) -> (w553:string[][])
              }
            }
          }
          frame True {
          }
        }
        n322 = Array Size(array=w500) -> (size(s)=w514:i32[])
        n323 = Index Array(array=w514) -> (element=w513:i32)  [unwired: 1 in]
        n324 = Decrement(x=w513) -> (x-1=w498:i32)
        n325 = Delete From Array(array=w500, index (row)=w498) -> (array with subset deleted=w497:string[][])  [unwired: 2 in, 1 out]
        n326 = Index Array(array=w497, index (col) #1=2 ("disabled index (col)"), index (col) #2=3 ("index (col)"), index (col) #3=4 ("index (col)")) -> (element #1=w511:string[], element #2=w503:string[], element #3=w501:string[])  [unwired: 3 in]
        n327 = local write "Input_Table"(w500) -> ()
        n328 = for {
          tunnel: w501 -> [w529] mode=indexing
          tunnel: T7 {"use custom"=FALSE, "lin/log"=0, "unit"="", "dB ref"=0.0, "common dB"=0} ("Custom unit info") -> [w535]
          tunnel: [w527] -> w508 mode=indexing
          w530 = "dB" ("x")
          n329 = Equal?(x=w530, y=w529) -> (x = y?=w531:bool)
          n330 = Select(t=w530, s=w531, f=w529) -> (s? t:f=w528:string)
          n331 = Select(t=u16 0 ("lin/log"), s=w531, f=u16 1) -> (s? t:f=w532:u16)
          n332 = Bundle By Name(cluster=w535, "lin/log"=w532, "unit"=w528) -> (w527:T7)
        }
        n333 = for {
          tunnel: w511 -> [w537] mode=indexing
          tunnel: [w536] -> w510 mode=indexing
          n334 = case shown="\"z\"" w537 {
            tunnel: [0 ("disabled index (col)") 1 ("disabled index (col)") 2 ("disabled index (col)")] -> w536
            frame "x", Default {
            }
            frame "y" {
            }
            frame "z" {
            }
          }
        }
        n335 = local read "User Equation Cluster"() -> (w516:T3)
        n336 = Bundle By Name(cluster=w516, "Input axis"=w510, "Input Values"=w503, "Custom unit input array"=w508) -> (w515:T3)
        n337 = property on="User Equation Cluster" class="Clust (strict)"("Val(Sgnl)"=w515) -> ()  [unwired: 2 in, 2 out]
      }
      event "Unit_in": Mouse Down {
        w586 = FALSE ("Unit")
        n338 = event-data() -> ()  [unwired: 1 in, 7 out]
        n339 = local read "User Equation Cluster"() -> (w582:T3)
        n340 = local read "Input_Table"() -> (w583:string[][])
        n341 = local read "Row_unit"() -> (w577:i32)
        n342 = Unbundle By Name(w582) -> ("Custom unit input array"=w581:T9)
        n343 = local write "Unit_in"(w586) -> ()
        n344 = property on="Unit_in" class="Bool (strict)"("Visible"=w586) -> ()  [unwired: 2 in, 2 out]
        n345 = Replace Array Subset(array=w583, new element="Unit..." ("element"), index (row)=w577, index (col)=5 ("disabled index (col)")) -> (w576:string[][])
        n346 = Index Array(array=w583, index (row)=w577, index (col)=4 ("disabled index (col)")) -> (element=w579:string)
        n347 = Index Array(array=w583, index (row)=w577, index (col)=0 ("disabled index (col)")) -> (element=w589:string)
        n348 = Equal?(x=w589, y="User Defined Constant") -> (x = y?=w578:bool)
        n349 = Index Array(array=w581, index=w577) -> (element=w580:T7)
        n350 = case shown="False" w578 {
          tunnel: w579 -> [_ w623]
          tunnel: w577 -> [_ w600]
          tunnel: w576 -> [w596 w621]
          tunnel: [w596 w619] -> w575
          tunnel: w582 -> [_ w614]
          tunnel: w580 -> [_ w608]
          tunnel: w581 -> [_ w601]
          frame False {
            n351 = call "CRYGet Error Message.vi"("Error No"=12, "Kind"="Post Processing") -> ("Message Sub 3"=w592:string, "Window Title"=w593:string)  [unwired: 4 in, 4 out]
            n352 = call "CRYMessage Dialog.vi"("Window Title"=w593, "YesNoCancel"=T8."OK", "Message Content"=w592) -> ()  [unwired: 7 in, 2 out]
          }
          frame True {
            n353 = Unbundle By Name(w608) -> ("lin/log"=w613:u16, "unit"=w612:string, "dB ref"=w611:dbl, "common dB"=w610:u16)
            n354 = call "CRYUnits setup.vi"("Scale visible?"=TRUE, "dB/Lin"=w613, "Unit:"=w612, "dB ref:"=w611, "Common dB ref."=w610) -> ("New Scale"=w606:u16, "New unit Lin"=w605:string, "New dB ref"=w604:dbl, "Common dB #"=w603:u16, "Use custom unit out"=w607:bool, "Cancelled?"=w609:bool)  [unwired: 3 in, 2 out]
            n355 = Bundle By Name(cluster=w608, "use custom"=w607, "lin/log"=w606, "unit"=w605, "dB ref"=w604, "common dB"=w603) -> (w602:T7)
            n356 = Equal To 0?(x=w606) -> (x = 0?=w618:bool)
            n357 = Select(t=w623, s=w609, f=w605) -> (s? t:f=w617:string)
            n358 = Select(t=w608, s=w609, f=w602) -> (s? t:f=w599:T7)
            n359 = Select(t="dB", s=w618, f=w617) -> (s? t:f=w615:string)
            n360 = Replace Array Subset(array=w621, new element=w615, index (row)=w600, index (col)=4 ("disabled index (col)")) -> (w619:string[][])
            n361 = Replace Array Subset(array=w601, new element=w599, index=w600) -> (w598:T9)
            n362 = Bundle By Name(cluster=w614, "Custom unit input array"=w598) -> (w620:T3)
            n363 = property on="User Equation Cluster" class="Clust (strict)"("Val(Sgnl)"=w620) -> ()  [unwired: 2 in, 2 out]
          }
        }
        n364 = local write "Input_Table"(w575) -> ()
      }
      event "Result_Table": Mouse Down {
        w627 = 5 ("y")
        n365 = event-data() -> ("Coords"=w636:T10)  [unwired: 1 in, 6 out]
        n366 = invoke on="Result_Table" class="Tbl (strict)" method="Point To Row Column"("Point"=w636) -> ("CellPosition"=w630:T4)  [unwired: 5 in, 5 out]
        n367 = local read "Result_Table"() -> (w628:string[][])
        n368 = Unbundle By Name(w630) -> ("Row"=w629:i32, "Column"=w634:i32)
        n369 = property on="Unit_res" class="Bool (strict)"() -> ("Visible"=w635:bool)  [unwired: 2 in, 2 out]
        n370 = Not(x=w635) -> (.not. x?=w632:bool)
        n371 = Equal?(x=w634, y=w627) -> (x = y?=w633:bool)
        n372 = Index Array(array=w628, index (row)=w629, index (col)=w627) -> (element=w626:string)
        n373 = Not Equal?(x="", y=w626) -> (x != y?=w624:bool)
        n374 = Compound Arithmetic op=AND(w633, w624, w632) -> (w631:bool)
        n375 = case shown="True" w631 {
          tunnel: w630 -> [_ w652]
          tunnel: w629 -> [_ w646]
          frame False {
            n376 = property on="Unit_res" class="Bool (strict)"("Visible"=FALSE) -> ()  [unwired: 2 in, 2 out]
          }
          frame True {
            w642 = FALSE ("Unit")
            w644 = u32 3 ("y")
            n377 = property on="Result_Table" class="Tbl (strict)"("Active Cell"=w652) -> ("Cell Size"=w650:T11, "ActiveCellPos"=w654:T12)  [unwired: 2 in, 2 out]
            n378 = Unbundle By Name(w650) -> ("Width"=w640:u32, "Height"=w648:u32)
            n379 = Unbundle By Name(w654) -> ("Left"=w655:i32, "Top"=w645:i32)
            n380 = Add(x=u32 2, y=w640) -> (x+y=w638:u32)
            n381 = Add(x=w648, y=w644) -> (x+y=w649:u32)
            n382 = Subtract(x=w645, y=w644) -> (x-y=w643:u32)
            n383 = Decrement(x=w655) -> (x-1=w641:i32)
            n384 = Bundle(w638, w649) -> (w647:cluster{u32, u32})  [unwired: 1 in]
            n385 = Bundle(w641, w643) -> (w651:cluster{i32, u32})  [unwired: 1 in]
            n386 = property on="Unit_res" class="Bool (strict)"("Value"=w642, "Visible"=TRUE, "Button Size"=w647, "Position"=w651) -> ()  [unwired: 2 in, 2 out]
            n387 = property on="Unit_in" class="Bool (strict)"("Visible"=w642) -> ()  [unwired: 2 in, 2 out]
            "Row_unit res" <- w646
          }
        }
      }
      event "Unit_res": Mouse Down {
        w687 = FALSE ("Unit")
        n388 = event-data() -> ()  [unwired: 1 in, 7 out]
        n389 = local read "User Equation Cluster"() -> (w660:T3)
        n390 = local read "Row_unit res"() -> (w658:i32)
        n391 = local read "Result_Table"() -> (w659:string[][])
        n392 = Unbundle By Name(w660) -> ("Custom unit results array"=w664:T9)
        n393 = local write "Unit_res"(w687) -> ()
        n394 = property on="Unit_res" class="Bool (strict)"("Visible"=w687) -> ()  [unwired: 2 in, 2 out]
        n395 = Replace Array Subset(array=w659, new element="Unit..." ("element"), index (row)=w658, index (col)=5 ("disabled index (col)")) -> (w682:string[][])
        n396 = Index Array(array=w659, index (row)=w658, index (col)=4 ("disabled index (col)")) -> (element=w685:string)
        n397 = Index Array(array=w664, index=w658) -> (element=w671:T7)
        n398 = Unbundle By Name(w671) -> ("lin/log"=w676:u16, "unit"=w673:string, "dB ref"=w674:dbl, "common dB"=w675:u16)
        n399 = call "CRYUnits setup.vi"("Scale visible?"=TRUE, "dB/Lin"=w676, "Unit:"=w673, "dB ref:"=w674, "Common dB ref."=w675) -> ("New Scale"=w667:u16, "New unit Lin"=w668:string, "New dB ref"=w669:dbl, "Common dB #"=w670:u16, "Use custom unit out"=w666:bool, "Cancelled?"=w672:bool)  [unwired: 3 in, 2 out]
        n400 = Bundle By Name(cluster=w671, "use custom"=w666, "lin/log"=w667, "unit"=w668, "dB ref"=w669, "common dB"=w670) -> (w665:T7)
        n401 = Equal To 0?(x=w667) -> (x = 0?=w680:bool)
        n402 = Select(t=w685, s=w672, f=w668) -> (s? t:f=w678:string)
        n403 = Select(t=w671, s=w672, f=w665) -> (s? t:f=w663:T7)
        n404 = Select(t="dB", s=w680, f=w678) -> (s? t:f=w677:string)
        n405 = Replace Array Subset(array=w682, new element=w677, index (row)=w658, index (col)=4 ("disabled index (col)")) -> (w656:string[][])
        n406 = Replace Array Subset(array=w664, new element=w663, index=w658) -> (w662:T9)
        n407 = local write "Result_Table"(w656) -> ()
        n408 = Bundle By Name(cluster=w660, "Custom unit results array"=w662) -> (w657:T3)
        n409 = property on="User Equation Cluster" class="Clust (strict)"("Val(Sgnl)"=w657) -> ()  [unwired: 2 in, 2 out]
      }
      event "Input_Table": Value Change {
        n410 = event-data() -> ()  [unwired: 1 in, 5 out]
        n411 = local read "User Equation Cluster"() -> (w697:T3)
        n412 = local read "Input_Table"() -> (w717:string[][])
        n413 = Unbundle By Name(w697) -> ("Input Values"=w700:string[])
        n414 = Index Array(array=w717, index (col) #1=0 ("disabled index (col)"), index (col) #2=1 ("index (col)"), index (col) #3=2 ("index (col)"), index (col) #4=3 ("index (col)"), index (col) #5=5 ("index (col)")) -> (element #1=w716:string[], element #2=w712:string[], element #3=w709:string[], element #4=w701:string[], element #5=w695:string[])  [unwired: 5 in]
        n415 = for {
          tunnel: w716 -> [w754] mode=indexing
          tunnel: [w767] -> w714 mode=indexing
          tunnel: w712 -> [w758] mode=indexing
          tunnel: w712 -> [w762]
          tunnel: [w757] -> w711 mode=indexing
          tunnel: w709 -> [w756] mode=indexing
          tunnel: [w750] -> w708 mode=indexing
          tunnel: [w755] -> w704 mode=indexing
          tunnel: "User Defined Constant" -> [w753]
          tunnel: w701 -> [w748] mode=indexing
          tunnel: w700 -> [w747] mode=indexing
          tunnel: [w746] -> w699 mode=indexing
          tunnel: w695 -> [w742] mode=indexing
          tunnel: [w741] -> w693 mode=indexing
          n416 = Equal?(x=w754, y=w753) -> (x = y?=w749:bool)
          n417 = for {
            tunnel: w762 -> [w778] mode=indexing
            tunnel: [w775] -> w764 mode=indexing
            n418 = Match Pattern(string=w778, regular expression="a") -> (after substring=w776:string)  [unwired: 1 in, 3 out]
            n419 = Decimal String To Number(string=w776) -> (number=w775:i32)  [unwired: 2 in, 1 out]
          }
          n420 = Equal?(x=w742, y="") -> (x = y?=w744:bool)
          n421 = Equal?(x=w758, y="") -> (x = y?=w759:bool)
          n422 = Select(t="Unit..." ("element"), s=w744, f=w742) -> (s? t:f=w741:string)
          n423 = case shown="Default" w756 {
            selector: w756 -> [_ w774]
            tunnel: ["y" w774] -> w752
            frame Default {
            }
            frame "'y'", "'z'", "x" {
            }
          }
          n424 = Select(t=w748, s=w749, f=w747) -> (s? t:f=w746:string)
          n425 = Array Max & Min(array=w764) -> (max value=w763:i32)  [unwired: 3 out]
          n426 = Increment(x=w763) -> (x+1=w761:i32)
          n427 = Select(t="y", s=w749, f=w752) -> (s? t:f=w750:string)
          n428 = Equal?(x=w754, y="") -> (x = y?=w768:bool)
          n429 = Number To Decimal String(number=w761) -> (decimal integer string=w760:string)  [unwired: 1 in]
          n430 = case shown="\"x\", Default" w750 {
            tunnel: [0 ("disabled index (col)") 1 ("disabled index (col)") 2 ("disabled index (col)")] -> w755
            frame "x", Default {
            }
            frame "y" {
            }
            frame "z" {
            }
          }
          n431 = Select(t="<Select Operand>", s=w768, f=w754) -> (s? t:f=w767:string)
          n432 = Select(t=w760, s=w759, f=w758) -> (s? t:f=w757:string)
        }
        n433 = Unbundle By Name(w697) -> ("Custom unit input array"=w723:T9)
        n434 = for {
          tunnel: w723 -> [w784] mode=indexing
          tunnel: [w779] -> w692 mode=indexing
          n435 = Unbundle By Name(w784) -> ("lin/log"=w783:u16, "unit"=w781:string)
          n436 = Equal To 0?(x=w783) -> (x = 0?=w782:bool)
          n437 = Select(t="dB", s=w782, f=w781) -> (s? t:f=w779:string)
        }
        n438 = Array Size(array=w692) -> (size(s)=w691:i32)
        n439 = Replace Array Subset(array=w717, new element #1=w714, index (col) #1=0 ("disabled index (col)"), new element #2=w711, index (col) #2=1 ("index (col)"), new element #3=w708, index (col) #3=2 ("index (col)"), new element #4=w699, index (col) #4=3 ("index (col)"), new element #5=w692, index (col) #5=4 ("index (col)"), new element #6=w693, index (col) #6=5 ("index (col)")) -> (w690:string[][])  [unwired: 6 in]
        n440 = Increment(x=w691) -> (x+1=w689:i32)
        n441 = for {
          N: w689 -> [_]
          tunnel: w690 -> [w730] mode=indexing
          tunnel: w689 -> [w728]
          tunnel: [w727] -> w688 mode=indexing
          i -> [w729]
          n442 = for {
            tunnel: w730 -> [w733] mode=indexing
            tunnel: w729 -> [w739]
            tunnel: w728 -> [w738]
            tunnel: [w731] -> w727 mode=indexing
            i -> [w740]
            n443 = Decrement(x=w738) -> (x-1=w737:i32)
            n444 = Not Equal To 0?(x=w740) -> (x != 0?=w735:bool)
            n445 = Equal?(x=w737, y=w739) -> (x = y?=w736:bool)
            n446 = And(x=w736, y=w735) -> (x .and. y?=w734:bool)
            n447 = Select(t="", s=w734, f=w733) -> (s? t:f=w731:string)
          }
        }
        n448 = Index Array(array=w688, index (col) #1=0 ("disabled index (col)"), index (col) #2=1 ("index (col)"), index (col) #3=3 ("index (col)")) -> (element #1=w720:string[], element #2=w706:string[], element #3=w698:string[])  [unwired: 3 in]
        n449 = local write "Input_Table"(w688) -> ()
        n450 = Bundle By Name(cluster=w697, "Input Curve Names"=w720, "Input Curve Variables"=w706, "Input axis"=w704, "Input Values"=w698) -> (w719:T3)
        n451 = property on="User Equation Cluster" class="Clust (strict)"("Val(Sgnl)"=w719) -> ()  [unwired: 2 in, 2 out]
      }
      event "Result_Table": Value Change {
        n452 = event-data() -> ()  [unwired: 1 in, 5 out]
        n453 = local read "User Equation Cluster"() -> (w790:T3)
        n454 = local read "Result_Table"() -> (w791:string[][])
        n455 = Unbundle By Name(w790) -> ("Desired Result Variables"=w789:string[], "Results axis"=w809:u16[], "Result Values"=w805:string[], "Custom unit results array"=w803:T9)
        n456 = Index Array(array=w791, index (col)=0 ("disabled index (col)")) -> (element=w798:string[])  [unwired: 1 in]
        n457 = Index Array(array=w791, index (col)=5 ("disabled index (col)")) -> (element=w794:string[])  [unwired: 1 in]
        n458 = for {
          tunnel: w803 -> [w830] mode=indexing
          tunnel: [w825] -> w788 mode=indexing
          n459 = Unbundle By Name(w830) -> ("lin/log"=w829:u16, "unit"=w827:string)
          n460 = Equal To 0?(x=w829) -> (x = 0?=w828:bool)
          n461 = Select(t="dB", s=w828, f=w827) -> (s? t:f=w825:string)
        }
        n462 = for {
          tunnel: w809 -> [w832] mode=indexing
          tunnel: [w831] -> w807 mode=indexing
          n463 = case shown="1" w832 {
            tunnel: ["x" "y" "z"] -> w831
            frame 0, Default {
            }
            frame 1 {
            }
            frame 2 {
            }
          }
        }
        n464 = for {
          tunnel: w794 -> [w814] mode=indexing
          tunnel: [w813] -> w792 mode=indexing
          n465 = Equal?(x=w814, y="") -> (x = y?=w815:bool)
          n466 = Select(t="Unit..." ("element"), s=w815, f=w814) -> (s? t:f=w813:string)
        }
        n467 = for {
          tunnel: w798 -> [w818] mode=indexing
          tunnel: w791 -> [w822]
          tunnel: [w817] -> w797 mode=indexing
          i -> [w820]
          n468 = Index Array(array=w822, index (row)=w820, index (col)=1 ("disabled index (col)")) -> (element=w819:string)
          n469 = Equal?(x=w818, y="") -> (x = y?=w823:bool)
          n470 = Select(t=w819, s=w823, f=w818) -> (s? t:f=w817:string)
        }
        n471 = Replace Array Subset(array=w791, new element #1=w797, index (col) #1=0 ("disabled index (col)"), new element #2=w789, index (col) #2=1 ("disabled index (col)"), new element #3=w807, index (col) #3=2 ("index (col)"), new element #4=w805, index (col) #4=3 ("index (col)"), new element #5=w788, index (col) #5=4 ("index (col)"), new element #6=w792, index (col) #6=5 ("index (col)")) -> (w786:string[][])  [unwired: 6 in]
        n472 = Array Size(array=w788) -> (size(s)=w787:i32)
        n473 = for {
          N: w787 -> [_]
          tunnel: w786 -> [w811] mode=indexing
          tunnel: [w811] -> w785 mode=indexing
        }
        n474 = Index Array(array=w785, index (col)=0 ("disabled index (col)")) -> (element=w801:string[])  [unwired: 1 in]
        n475 = local write "Result_Table"(w785) -> ()
        n476 = Bundle By Name(cluster=w790, "Desired Result Names"=w801) -> (w800:T3)
        n477 = property on="User Equation Cluster" class="Clust (strict)"("Val(Sgnl)"=w800) -> ()  [unwired: 2 in, 2 out]
      }
      event "Res_Table Change": Value Change {
        n478 = event-data() -> ()  [unwired: 1 in, 5 out]
        n479 = local read "String Ref Out"() -> (w846:refnum<vi>)
        n480 = local write "Res_Table Change"(FALSE ("Table Change")) -> ()
        n481 = property class="Str"(reference=w846) -> ("Value"=w845:string)  [unwired: 1 in, 2 out]
        n482 = call "CRYUnflatten User Equation Cluster.vi"("Flatten user equation cluster string"=w845) -> ("User Equation Cluster"=w844:T3)  [unwired: 8 in, 2 out]
        n483 = Unbundle By Name(w844) -> ("Desired Result Names"=w840:string[], "Desired Result Variables"=w839:string[], "Result Values"=w838:string[], "Custom unit results array"=w837:T9)
        n484 = local write "User Equation Cluster"(w844) -> ()
        n485 = Array Size(array=w840) -> (size(s)=w843:i32)
        n486 = Equal To 0?(x=w843) -> (x = 0?=w841:bool)
        n487 = case shown="False" w841 {
          tunnel: w839 -> [w861 _]
          tunnel: w838 -> [w858 _]
          tunnel: [w854 w868] -> w836
          tunnel: string[][] [] ("Result Table") -> [w853 w868]
          tunnel: w840 -> [w852 _]
          tunnel: w837 -> [w849 _]
          frame False {
            n488 = for {
              tunnel: w849 -> [w867] mode=indexing
              tunnel: [w862] -> w848 mode=indexing
              n489 = Unbundle By Name(w867) -> ("lin/log"=w866:u16, "unit"=w864:string)
              n490 = Equal To 0?(x=w866) -> (x = 0?=w865:bool)
              n491 = Select(t="dB", s=w865, f=w864) -> (s? t:f=w862:string)
            }
            n492 = Array Size(array=w861) -> (size(s)=w857:i32)
            n493 = Initialize Array("y", w857) -> (w859:string[])
            n494 = Initialize Array("Unit..." ("element"), w857) -> (w855:string[])
            n495 = Build Array(w852, w861, w859, w858, w848, w855) -> (w851:string[][])
            n496 = Transpose 2D Array(2D array=w851) -> (transposed array=w850:string[][])
            n497 = Insert Into Array(array=w853, new element=w850) -> (w854:string[][])  [unwired: 2 in]
          }
          frame True {
          }
        }
        n498 = local write "Result_Table"(w836) -> ()
      }
      event "In_Table Change": Value Change {
        n499 = event-data() -> ("NewVal"=w886:i32)  [unwired: 1 in, 4 out]
        n500 = local read "Input_Table"() -> (w869:string[][])
        n501 = Delete From Array(array=w869, index (row)=w886) -> (array with subset deleted=w870:string[][])  [unwired: 2 in, 1 out]
        n502 = local write "Input_Table"(w870) -> ()
        n503 = Index Array(array=w870, index (col) #1=0 ("disabled index (col)"), index (col) #2=1 ("index (col)"), index (col) #3=2 ("index (col)"), index (col) #4=3 ("index (col)"), index (col) #5=4 ("index (col)")) -> (element #1=w879:string[], element #2=w877:string[], element #3=w875:string[], element #4=w873:string[], element #5=w871:string[])  [unwired: 5 in]
        n504 = for {
          tunnel: w875 -> [w897] mode=indexing
          tunnel: [w896] -> w882 mode=indexing
          n505 = case shown="\"x\", Default" w897 {
            tunnel: [0 ("disabled index (col)") 1 ("disabled index (col)") 2 ("disabled index (col)")] -> w896
            frame "x", Default {
            }
            frame "y" {
            }
            frame "z" {
            }
          }
        }
        n506 = for {
          tunnel: w871 -> [w889] mode=indexing
          tunnel: T7 {"use custom"=FALSE, "lin/log"=0, "unit"="", "dB ref"=0.0, "common dB"=0} ("Custom unit info") -> [w895]
          tunnel: [w887] -> w880 mode=indexing
          w890 = "dB" ("x")
          n507 = Equal?(x=w890, y=w889) -> (x = y?=w891:bool)
          n508 = Select(t=w890, s=w891, f=w889) -> (s? t:f=w888:string)
          n509 = Select(t=u16 0 ("lin/log"), s=w891, f=u16 1) -> (s? t:f=w892:u16)
          n510 = Bundle By Name(cluster=w895, "lin/log"=w892, "unit"=w888) -> (w887:T7)
        }
        n511 = local read "User Equation Cluster"() -> (w885:T3)
        n512 = Bundle By Name(cluster=w885, "Input Curve Names"=w879, "Input Curve Variables"=w877, "Input axis"=w882, "Input Values"=w873, "Custom unit input array"=w880) -> (w884:T3)
        n513 = property on="User Equation Cluster" class="Clust (strict)"("Val(Sgnl)"=w884) -> ()  [unwired: 2 in, 2 out]
      }
      event "Clear All": Value Change {
        w907 = ""
        w905 = string[][] [] ("Result Table")
        n514 = event-data() -> ()  [unwired: 1 in, 5 out]
        n515 = local write "Clear All"(FALSE ("Clear All")) -> ()
        n516 = Build Array("<Select Operand>", w907, w907, w907, w907, w907) -> (w902:string[])
        n517 = Insert Into Array(array=w905, index (row)=0, new element=w902) -> (w904:string[][])  [unwired: 1 in]
        n518 = local write "Result_Table"(w905) -> ()
        n519 = local write "Input_Table"(w904) -> ()
        n520 = property on="User Equation Cluster" class="Clust (strict)"("Val(Sgnl)"=T3 {"Custom unit input array"=[], "Custom unit results array "=[], "Desired Result Variables"=[], "Desired Result Names"=[], "Input Curve Names"=[], "Input Curve Variables"=[], "equation"="", "Input axis"=[], "Results axis"=[], "# input curves"=0, "# Desired result curves "=0, "Input Values"=[], "Result Values"=[]} ("Value (Signaling)")) -> ()  [unwired: 2 in, 2 out]
      }
      event "CurLibChange": Value Change {
        n521 = event-data() -> ()  [unwired: 1 in, 6 out]
        n522 = call "CRYGet Current TS Steps.vi"() -> ("SelectStepNumber in Tree"=w918:i32, "Steps"=w919:T6[])  [unwired: 7 in, 3 out]
        n523 = Index Array(array=w919, index=w918) -> (element=w920:T6)
        n524 = local read "On/Off Line"() -> (w923:bool)
        n525 = Unbundle By Name(w920) -> ("No.VI"=w915:i32)
        n526 = case shown="True" w923 {
          tunnel: enum16{"Curves", "Values", "Results", "WFM"}."Values" ("Type In") -> [w925 w932]
          tunnel: enum16{"Curves", "Values", "Results", "WFM"}."Curves" ("Type In") -> [w926 w931]
          tunnel: w915 -> [_ w930]
          tunnel: [w927 w929] -> w921
          tunnel: [w924 w928] -> w922
          frame False {
            n527 = call "CRYGet Curve Library Array.vi"("Type In"=w925) -> ("Curve/Value array"=w924:T1)  [unwired: 10 out]
            n528 = call "CRYGet Curve Library Array.vi"("Type In"=w926) -> ("Curve/Value array"=w927:T1)  [unwired: 10 out]
          }
          frame True {
            n529 = call "CRYGet Upper Step Data.vi"("Type In"=w931, "No.VI"=w930) -> ("Curve array"=w929:T1)  [unwired: 9 out]
            n530 = call "CRYGet Upper Step Data.vi"("Type In"=w932, "No.VI"=w930) -> ("Value array"=w928:T1)  [unwired: 9 out]
          }
        }
        n531 = Build Array (concatenate)(w921, w922) -> (w910:T1)
        n532 = local write "Curves&Values"(w910) -> ()
        n533 = for {
          tunnel: w910 -> [w934] mode=indexing
          tunnel: [w933] -> w909 mode=indexing
          n534 = Unbundle By Name(w934) -> ("Name"=w933:string)
        }
        n535 = local write "DataNames"(w909) -> ()
        n536 = Build Array (concatenate)("<Select Operand>", w909, "User Defined Constant", "Remove this Item") -> (w911:string[])
        n537 = property on="Ope_Ring" class="Ring (strict)"("Strings []"=w911) -> ()  [unwired: 2 in, 2 out]
      }
    }
    n538 = global read "CRYMain Sub Window Global.vi" "gStop"() -> (w64:bool)
    n539 = Or(x="stop", y=w64) -> (x .or. y?=w62:bool)
    n540 = control-ref of="This VI"() -> (w61:refnum<vi>)
  }
  n541 = property class="VI"(reference=w2, "Front Panel.Open"=FALSE ("Front Panel Window:Open")) -> ()  [unwired: 1 in, 2 out]
